vi "Pre Launch Init.vi"(11 "Remote Operation Abstract in":refnum<class "Remote Operation Abstract.lvclass">) -> (0 "error out":errorcluster, 3 "Remote Operation Abstract out":refnum<class "Remote Operation Abstract.lvclass">)   [LabVIEW 2018, in "Remote Operation Abstract.lvlib" / "Remote Operation Abstract.lvclass"]
doc: "(<B>Filename</B>: Actor Framework.lvlib:Actor.lvclass:Pre Launch Init.vi)\n\nDefines behavior that occurs after the Launch Nested Actor method is invoked but before the actor's Actor Core method begins running.\n\nBy default, this method does nothing. A descendant class may override it to define behavior."
uses:
  Remote Operation Abstract.lvclass
  Remote Operation Abstract.lvclass/Remote Operation Abstract.ctl
  EMS Generic Actor/EMS Generic/EMS Generic.lvclass
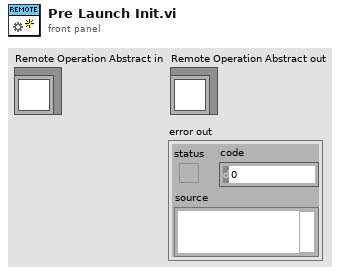
[diagram p1: front panel]
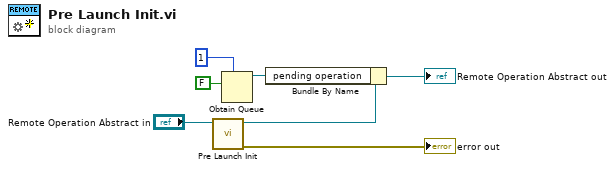
[diagram p0: block diagram]
diagram:
  n1 = call-parent "Pre Launch Init.vi"("EMS Generic in"="Remote Operation Abstract in") -> ("error out"=→"error out":errorcluster, "EMS Generic out"=w6:refnum<class "Remote Operation Abstract.lvclass">)  [unwired: 9 in]
  n2 = Obtain Queue(max queue size (-1, unlimited)=1, element data type=FALSE) -> (queue out=w1:refnum<queue>)  [unwired: 3 in, 2 out]
  n3 = Bundle By Name(cluster=w6, "pending operation"=w1) -> (→"Remote Operation Abstract out":refnum<class "Remote Operation Abstract.lvclass">)
